vi "Restarts Loop to Main.vi"(0 "Actual Pump Starts":u32[](array[numeric])=[0, 0, 0, 0, 0, 0], 1 "Cmd Pump Starts":u32[](array[numeric])=[0, 0, 0, 0, 0, 0], 2 "Pump No Starts":u32[](array[numeric])=[0, 0, 0, 0, 0, 0], 3 "Restarts":i32[](array[numeric])=[0, 0, 0, 0, 0, 0], 5 "Error IN":errorcluster, 8 "Write (F)":bool) -> (14 "Actual Pump Starts OUT":u32[](array[numeric]), 15 "Cmd Pump Starts OUT":u32[](array[numeric]), 16 "Pump No Starts OUT":u32[](array[numeric]), 17 "Restarts OUT":i32[](array[numeric]), 19 "Error OUT":errorcluster)   [LabVIEW 2019]
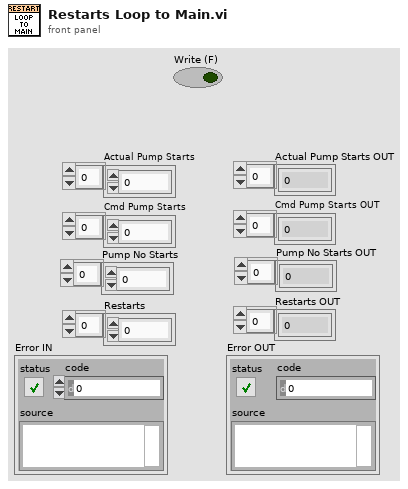
[diagram p1: front panel]
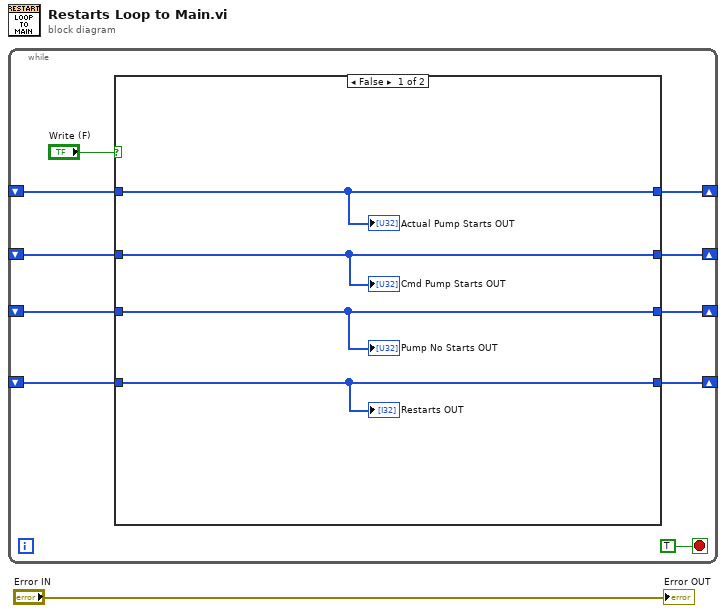
[diagram p0: block diagram]
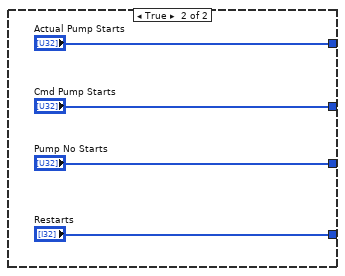
[diagram p2: hidden frame]
diagram:
  n1 = while {
    shift-right: [w9] -> _
    shift-left: _ -> [w7]
    shift-right: [w8] -> _
    shift-left: _ -> [w6]
    shift-right: [w5] -> _
    shift-left: _ -> [w4]
    shift-right: [w2] -> _
    shift-left: _ -> [w3]
    stop <- TRUE stop-if-true
    n2 = case shown="False" "Write (F)" {
      tunnel: [w15 "Actual Pump Starts"] -> w9
      tunnel: [w14 "Cmd Pump Starts"] -> w8
      tunnel: w7 -> [w15 _]
      tunnel: w6 -> [w14 _]
      tunnel: [w13 "Restarts"] -> w5
      tunnel: w4 -> [w13 _]
      tunnel: [w12 "Pump No Starts"] -> w2
      tunnel: w3 -> [w12 _]
      frame False {
        "Actual Pump Starts OUT" <- w15
        "Cmd Pump Starts OUT" <- w14
        "Restarts OUT" <- w13
        "Pump No Starts OUT" <- w12
      }
      frame True {
      }
    }
  }
  "Error OUT" <- "Error IN"
